vi "GT Get Dll Version.vi"(8 "error in (no error)":errorcluster caption="错误输入（无错误）", 11 "pDllVersion":string) -> (0 "error out":errorcluster caption="错误输出", 2 "function return":i16, 3 "pDllVersion out":string)   [LabVIEW 2020, in "gts.lvlib"]
doc: "GT_API GT_GetDllVersion(char **pDllVersion);"
uses:
  gts.lvlib
  dll/32bit/multi_card/gts.dll
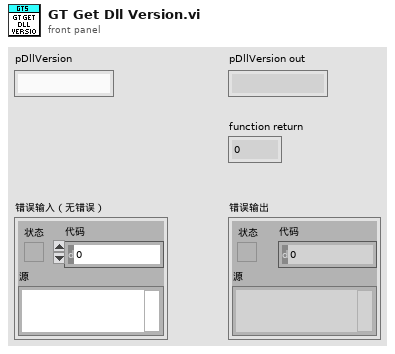
[diagram p1: front panel]
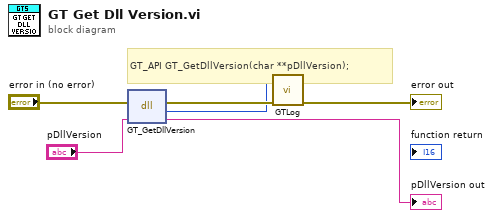
[diagram p0: block diagram]
diagram:
  # "GT_API GT_GetDllVersion(char **pDllVersion);"
  n1 = dll-call lib="C:/1228/dll/32bit/multi_card/gts.dll" fn="GT_GetDllVersion"(error in="error in (no error)", "pDllVersion"="pDllVersion") -> (error out=w3:errorcluster, w1:i16, "pDllVersion"=→"pDllVersion out":string)  [unwired: 2 in, 1 out]
  n2 = call "GTLog.vi"("error in (no error)"=w3, "Numeric"=w1) -> ("error out"=→"error out":errorcluster)  [unwired: 9 in]
